vi "GetVariableValues.vi"(8 "error in (no error)":errorcluster, 10 "SequenceStep":i32, 11 "VariableManagerRef in":refnum<vi>) -> (0 "error out":errorcluster, 2 "VariableValues":refnum<class "VariableValue.lvclass">[](array[class]), 3 "VariableManagerRef out":refnum<vi>)   [LabVIEW 2013, in "VariableManagerAPI.lvlib"]
doc: "Return variable values at the given sequence step, if SequenceStep is in the range [0, MaxSteps-1] \nReturn default variable values, if SequenceStepIn is outside the range [0, MaxSteps-1]\nSequenced variables is listed first.\n\nAn error is thrown if a sequence function cannot be evaluated."
uses:
  VariableManagerAPI.lvlib
  VariableManager/VariableManager.lvclass
  VariableValue/VariableValue.lvclass
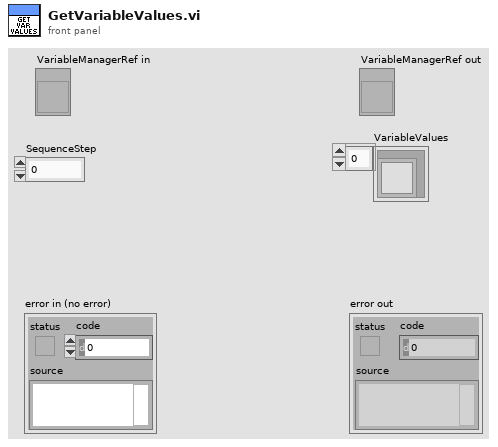
[diagram p1: front panel]
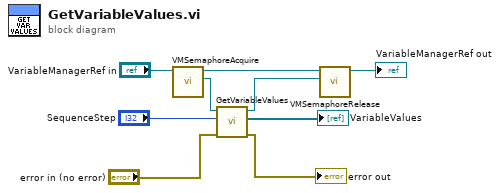
[diagram p0: block diagram]
diagram:
  n1 = call "VMSemaphoreAcquire.vi"("VariableManagerRef in"="VariableManagerRef in") -> ("VariableManager"=w6:refnum<class "VariableManager.lvclass">, "VariableManagerRef out"=w8:refnum<vi>)  [unwired: 7 in, 2 out]
  n2 = call-dynamic "GetVariableValues.vi"("error in (no error)"="error in (no error)", "SequenceStep"="SequenceStep", "VariablesManager in"=w6) -> ("error out"=→"error out":errorcluster, "VariableValues"=→"VariableValues":refnum<class "VariableValue.lvclass">[], "VariablesManager out"=w5:refnum<class "VariableManager.lvclass">)  [unwired: 6 in]
  n3 = call "VMSemaphoreRelease.vi"("VariableManager"=w5, "VariableManagerRef in"=w8) -> ("VariableManagerRef out"=→"VariableManagerRef out":refnum<vi>)  [unwired: 8 in, 1 out]
